vi "Initialize.vi"(8 "error in":errorcluster, 11 "VISA Interface in":refnum<class "VISA Interface.lvclass">) -> (0 "error out":errorcluster, 3 "VISA Interface out":refnum<class "VISA Interface.lvclass">)   [LabVIEW 2020, in "Plugin Instrument Driver.lvlib" / "VISA Interface.lvclass"]
doc: "Initialize VISA and Interface Settings."
uses:
  VISA Interface.lvclass
  builds/Libraries/Shared GUI Library.lvlibp/Shared GUI Library/Instrument Settings/Interface/Settings Container.ctl
  builds/Libraries/Shared GUI Library.lvlibp
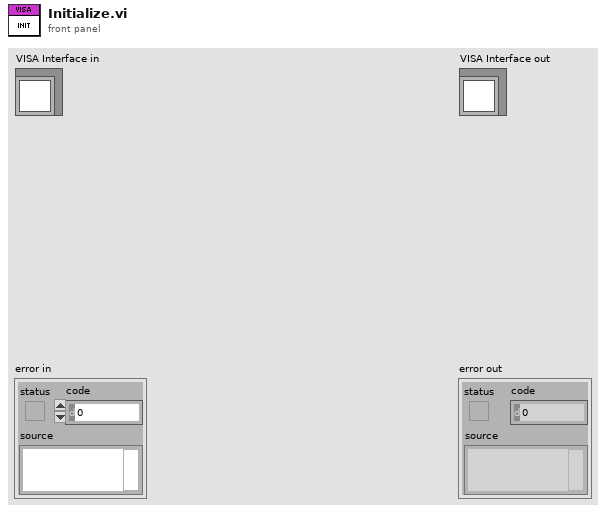
[diagram p1: front panel]
types:
  T1 = typedef "Shared GUI Library.lvlibp/Settings Container.ctl" = enum32{"GPIB", "VXI", "GPIB-VXI", "Serial", "PXI", "TCPIP", "USB", "FireWire", "Invalid"}
  T2 = typedef "Shared GUI Library.lvlibp/Serial Interafce.ctl" = cluster{"Baud Rate":u32, "Data Bits ":u16, "Parity":enum16{"None", "Odd", "Even"}, "Stop Bits":u16}
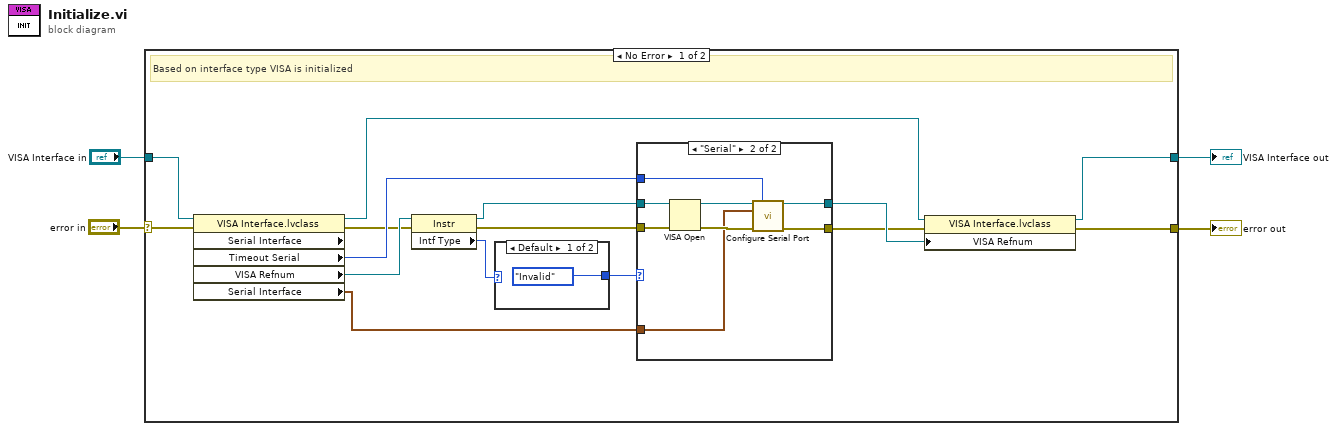
[diagram p0: block diagram]
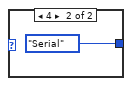
[diagram p2: hidden frame]
diagram:
  n1 = case shown="No Error" "error in" {
    selector: "error in" -> [w14 w33]
    tunnel: "VISA Interface in" -> [w15 w32]
    tunnel: [w7 w33] -> w2
    tunnel: [w6 w32] -> w1
    frame No Error {
      # "Based on interface type VISA is initialized"
      n2 = property class="VISA Interface.lvclass" props=["Serial Interface", "Timeout Serial", "VISA Refnum", "Serial Interface"](reference=w15, error in=w14) -> (reference out=w10:refnum<class "VISA Interface.lvclass">, error out=w11:errorcluster, "Timeout Serial"=w13:u32, "VISA Refnum"=w12:refnum<visa-resource-name>, "Serial Interface"=w5:T2)  [unwired: 1 out]
      n3 = property class="Instr"(reference=w12, error in=w11) -> (reference out=w17:refnum<visa-resource-name>, error out=w16:errorcluster, "Intf Type"=w19:u16)
      n4 = case shown="Default" w19 {
        tunnel: [Settings_Container."Invalid" ("Interface Type") Settings_Container."Serial" ("Interface Type")] -> w18
        frame Default {
        }
        frame 4 {
        }
      }
      n5 = case shown="\"Serial\"" w18 {
        tunnel: w16 -> [w23 w31]
        tunnel: w17 -> [w22 w30]
        tunnel: w13 -> [_ w29]
        tunnel: w5 -> [_ w26]
        tunnel: [w23 w25] -> w8
        tunnel: [w22 w24] -> w9
        frame "GPIB", Default {
        }
        frame "Serial" {
          n6 = VISA Open(error in (no error)=w31, VISA resource name=w30) -> (VISA resource name=w28:refnum<visa-resource-name>, error out=w27:errorcluster)  [unwired: 3 in]
          n7 = call "Configure Serial Port.vi"("VISA Refnum"=w28, "Timeout Serial"=w29, "Serial Interface"=w26, "error in"=w27) -> ("VISA resource name out"=w24:refnum<visa-resource-name>, "error out"=w25:errorcluster)  [unwired: 10 in]
        }
      }
      n8 = property class="VISA Interface.lvclass"(reference=w10, error in=w8, "VISA Refnum"=w9) -> (reference out=w6:refnum<class "VISA Interface.lvclass">, error out=w7:errorcluster)
    }
    frame Error {
    }
  }
  "error out" <- w2
  "VISA Interface out" <- w1
